vi "ODE Linear nth Order Numeric.vi"(0 "X0":dbl[](array[numeric]) format="%.2f", 1 "A (a0,a1,...an-1)":dbl[](array[numeric]) format="%.2f", 2 "number of points":u32=10, 3 "time start":dbl format="%.2f", 4 "time end":dbl=1.0 format="%.2f") -> (5 "Times":dbl[](array[numeric]) format="%.2f", 6 "X":dbl[](array[numeric]) format="%.2f", 7 "error":i32)   [LabVIEW 2020, in "NI_Gmath.lvlib"]
doc: "Solves an nth-order, homogeneous linear differential equation with constant coefficients in numeric form."
uses:
  NI_Gmath.lvlib
  Polynomial Roots (DBL).vi
  Solve Complex Linear Equations (single right hand).vi
  NI_AALPro.lvlib
  NI_AALBase.lvlib
panel:
  # "Example:\n\n A: 1.1 and 2.0 and -7.3 \n X0: 1.0 and 2.4 and -1.4 \n number of points: 100\n time start: 0.0 \n time end: 1.0"
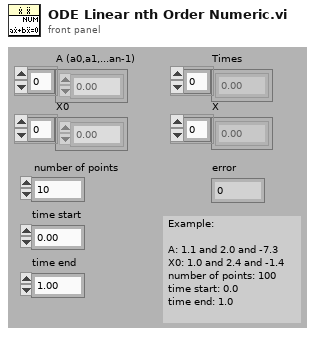
[diagram p1: front panel]
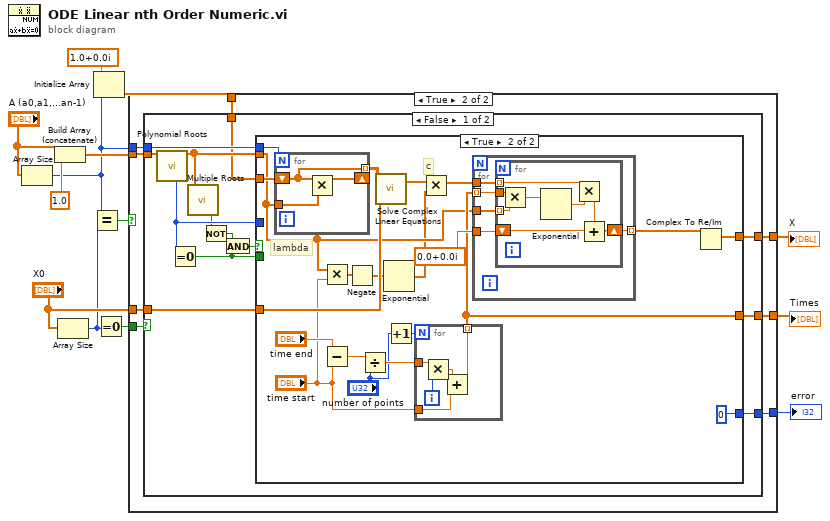
[diagram p0: block diagram]
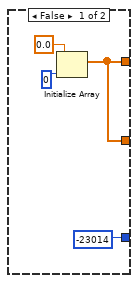
[diagram p2: hidden frame]
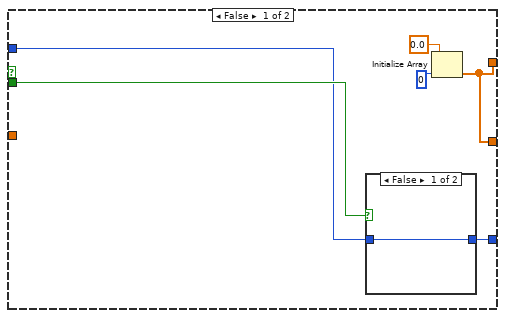
[diagram p3: hidden frame]
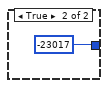
[diagram p4: hidden frame]
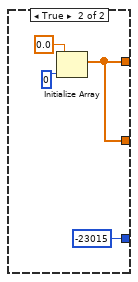
[diagram p5: hidden frame]
diagram:
  n1 = Array Size(array="A (a0,a1,...an-1)") -> (size(s)=w2:i32)
  n2 = Build Array (concatenate)("A (a0,a1,...an-1)", 1.0) -> (w8:dbl[])
  n3 = Array Size(array="X0") -> (size(s)=w9:i32)
  n4 = Equal?(x=w2, y=w9) -> (x = y?=w13:bool)
  n5 = Initialize Array(cdb 1.0+0.0i, w2) -> (w1:cdb[])
  n6 = Equal To 0?(x=w9) -> (x = 0?=w11:bool)
  n7 = case shown="True" w13 {
    tunnel: [-23014 w24] -> w12
    tunnel: w11 -> [_ w25]
    tunnel: w8 -> [_ w23]
    tunnel: "X0" -> [_ w22]
    tunnel: w2 -> [_ w21]
    tunnel: [w14 w20] -> w7
    tunnel: [w14 w19] -> w6
    tunnel: w1 -> [_ w18]
    frame False {
      n8 = Initialize Array(0.0, 0) -> (w14:dbl[])
    }
    frame True {
      n9 = case shown="False" w25 {
        tunnel: [w38 -23015] -> w24
        tunnel: w23 -> [w37 _]
        tunnel: w22 -> [w36 _]
        tunnel: w21 -> [w34 _]
        tunnel: [w33 w89] -> w20
        tunnel: [w32 w89] -> w19
        tunnel: w18 -> [w26 _]
        frame False {
          n10 = call-poly "Polynomial Roots.vi"("P(x)"=w37) -> ("error"=w35:i32, "Roots"=w31:cdb[])  [unwired: 9 in]
          n11 = Equal To 0?(x=w35) -> (x = 0?=w27:bool)
          n12 = call "Multiple Roots.vi"("Polynomial Roots"=w31) -> ("multiple roots"=w30:bool)
          n13 = Not(x=w30) -> (.not. x?=w29:bool)
          n14 = And(x=w29, y=w27) -> (x .and. y?=w28:bool)
          n15 = case shown="True" w28 {
            tunnel: w31 -> [_ w53]
            tunnel: w36 -> [_ w56]
            tunnel: [w39 0] -> w38
            tunnel: w35 -> [w40 _]
            tunnel: w34 -> [_ w61]
            tunnel: [w42 w58] -> w33
            tunnel: [w42 w57] -> w32
            tunnel: w27 -> [w41 _]
            tunnel: w26 -> [_ w55]
            frame False {
              n16 = case shown="False" w41 {
                tunnel: w40 -> [w45 _]
                tunnel: [w45 -23017] -> w39
                frame False {
                }
                frame True {
                }
              }
              n17 = Initialize Array(0.0, 0) -> (w42:dbl[])
            }
            frame True {
              # "lambda"
              # "C"
              n18 = for {
                N: w61 -> [_]
                tunnel: w53 -> [w88]
                shift-right: [w87] -> _
                shift-left: w55 -> [w86]
                tunnel: [w86] -> w54 mode=indexing
                n19 = Multiply(x=w86, y=w88) -> (x*y=w87:cdb[])
              }
              n20 = Multiply(x=w53, y="time start") -> (x*y=w51:cdb[])
              n21 = Subtract(x="time end", y="time start") -> (x-y=w65:dbl)
              n22 = Negate(x=w51) -> (-x=w50:cdb[])
              n23 = Divide(x=w65, y="number of points") -> (x/y=w64:dbl)
              n24 = call-poly "Solve Complex Linear Equations.vi"("Known Vector"=w56, "Input Matrix"=w54) -> ("Solution Vector"=w49:cdb[])  [unwired: 1 in, 1 out]
              n25 = Exponential(1:w50) -> (0:w48:cdb[])
              n26 = Increment(x="number of points") -> (x+1=w62:u32)
              n27 = for {
                N: w62 -> [_]
                tunnel: w64 -> [w85]
                tunnel: "time start" -> [w83]
                tunnel: [w81] -> w58 mode=indexing
                i -> [w84]
                n28 = Multiply(x=w85, y=w84) -> (x*y=w82:dbl)
                n29 = Add(x=w82, y=w83) -> (x+y=w81:dbl)
              }
              n30 = Multiply(x=w49, y=w48) -> (x*y=w47:cdb[])
              n31 = for {
                tunnel: w47 -> [w72]
                tunnel: cdb 0.0+0.0i -> [w71]
                tunnel: [w70] -> w59 mode=indexing
                tunnel: w58 -> [w69] mode=indexing
                tunnel: w53 -> [w68]
                n32 = for {
                  tunnel: w72 -> [w77] mode=indexing
                  shift-right: [w79] -> w70
                  shift-left: w71 -> [w80]
                  tunnel: w69 -> [w74]
                  tunnel: w68 -> [w73] mode=indexing
                  n33 = Multiply(x=w74, y=w73) -> (x*y=w75:cdb)
                  n34 = Exponential(1:w75) -> (0:w78:cdb)
                  n35 = Multiply(x=w77, y=w78) -> (x*y=w76:cdb)
                  n36 = Add(x=w76, y=w80) -> (x+y=w79:cdb)
                }
              }
              n37 = Complex To Re/Im(x + iy=w59) -> (x=w57:dbl[])  [unwired: 1 out]
            }
          }
        }
        frame True {
          n38 = Initialize Array(0.0, 0) -> (w89:dbl[])
        }
      }
    }
  }
  "error" <- w12
  "Times" <- w7
  "X" <- w6
